vi "Log Creation.vi"(8 "error in (no error)":errorcluster, 11 "CIFCorePlugin in":refnum<class "CIFCorePlugin.lvclass">) -> (0 "error out":errorcluster, 3 "CIFCorePlugin out":refnum<class "CIFCorePlugin.lvclass">)   [LabVIEW 2021, in "CIFCorePlugin.lvclass"]
uses:
  CIFCorePlugin.lvclass
  CIFUtilities/CIFLogs/Typedef/Plugin State Commands.ctl
  CIFCorePlugin.lvclass/CIFCorePlugin.ctl
  Accessors/Read Plugin Name.vi
  Accessors/Read gRPC Server Port.vi
  Accessors/Read Version.vi
  Accessors/Read Loader Name.vi
  CIFUtilities/CIFLogs/CIFLogs.lvlib
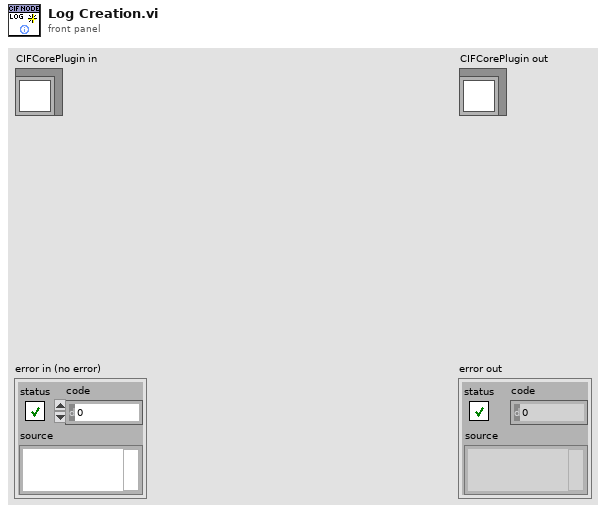
[diagram p1: front panel]
types:
  T1 = typedef "CIFLogs.lvlib/Plugin State Commands.ctl" = enum16{"Create", "Configure", "Run", "Pause", "Destroy", "Connect", "Force", "FIFO Instance"}
  T2 = typedef "CIFCoreCommon.lvlib/Version.ctl" = cluster{"Major":i32, "Minor":i32, "Fix":i32, "Build":i32}
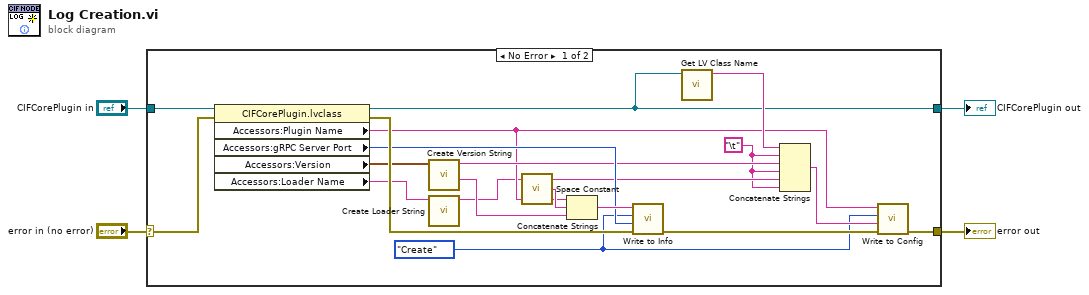
[diagram p0: block diagram]
diagram:
  n1 = case shown="No Error" "error in (no error)" {
    selector: "error in (no error)" -> [w21 w25]
    tunnel: [w8 w25] -> w3
    tunnel: [w10 w24] -> w1
    tunnel: "CIFCorePlugin in" -> [w23 w24]
    frame No Error {
      w5 = "\t"
      w6 = Plugin_State_Commands."Create" ("Command")
      n2 = property class="CIFCorePlugin.lvclass"(reference=w23, error in=w21) -> (reference out=w10:refnum<class "CIFCorePlugin.lvclass">, error out=w22:errorcluster, "Accessors:Plugin Name"=w11:string, "Accessors:gRPC Server Port"=w13:i32, "Accessors:Version"=w20:T2, "Accessors:Loader Name"=w18:string)
      n3 = call "Create Version String.vi"("Version"=w20) -> ("Version info string"=w19:string, "Version string"=w12:string)  [unwired: 9 in]
      n4 = call "Create Loader String.vi"("Loader Name"=w18) -> ("Loader string"=w7:string)  [unwired: 10 in]
      n5 = call <vilib>:"Space Constant.vi"() -> ("String"=w14:string)
      n6 = Concatenate Strings(w11, w14, w19) -> (w15:string)
      n7 = call "Write to Info.vi"("error in (no error)"=w22, "gRPC Port"=w13, "Command"=w6, "Plugin Name"=w15) -> ("error out"=w9:errorcluster)  [unwired: 7 in]
      n8 = call <vilib>:"Get LV Class Name.vi"("object"=w10) -> ("class name"=w16:string)  [unwired: 9 in, 1 out]
      n9 = Concatenate Strings(w16, w5, w12, w5, w7, w5) -> (w17:string)
      n10 = call "Write to Config.vi"("error in (no error)"=w9, "Additional Data"=w17, "Command"=w6, "Plugin Name"=w11) -> ("error out"=w8:errorcluster)  [unwired: 7 in]
    }
    frame Error {
    }
  }
  "error out" <- w3
  "CIFCorePlugin out" <- w1
